vi "PAM v1.3.vi"() -> ()   [LabVIEW 2011]
uses:
  PAM_Control.ctl
  <vilib>/Utility/error.llb/DialogType.ctl
  <vilib>/Analysis/Matrix/Datatypes/RealMatrix.ctl
  <vilib>/DAQmx/read.llb/DAQmx Read (Analog 1D Wfm NChan NSamp).vi
  <vilib>/DAQmx/write.llb/DAQmx Write (Analog 1D DBL NChan 1Samp).vi
  PAM SubVIs/RH Probe Global Var.vi
  <vilib>/DAQmx/configure/timing.llb/DAQmx Timing (Sample Clock).vi
  <vilib>/Utility/file.llb/Write To Spreadsheet File (string).vi
  <vilib>/Analysis/Matrix/Numeric/Conversions/Matrix To Array - RM.vi
  <vilib>/DAQmx/miscellaneous.llb/DAQmx Fill In Error Info.vi
  Program Files (x86)/National Instruments/LabVIEW 2011/resource/objmgr/daqmx.rc
  <vilib>/Analysis/Matrix/NI_Matrix.lvlib
panel:
  out "O3 Data":sgl[](graph)
  out "SO2 Data":sgl[](graph)
  out "NO, NO2, NOx Data":dbl[][](graph)
  out "Bad Advantech Data Points":dbl
  out "Run In Progress?":bool
  out "Manual":bool
  in  "MFC Sequence File":path=path "C:/Users/PAM/Dropbox/Research - Dr. Williams/PAM/LabVIEW PAM/PAM Edited/defaultMFCSequence.txt"
  out "Auto":bool
  out "P Unit":string
  out "Pressure Transducer":dbl(knob) scale=1.0004682058141296e-16..9998.829827870512
  out "Error Out":errorcluster
  out "Elapsed Time (min)":dbl format="%#_2g"
  in  "Run Start Time":timestamp format="%<%X\n%x>T"
  out "NOx Units":string="LPM"
  in  "NOx Control (LPM)":dbl(slide) scale=0.0..0.5
  out "NOx Reading (LPM) 3":dbl(slide) scale=0.0..0.5
  out "VOC Units":string="LPM"
  in  "VOC Control (LPM)":dbl(slide) scale=0.0..0.04
  out "VOC Reading (LPM)":dbl(slide) scale=0.0..0.04
  out "O2 Units":string="LPM"
  in  "O2 Control (LPM)":dbl(slide) scale=0.0..1.0
  out "O2 Reading (LPM)":dbl(slide) scale=0.0..1.0 scale format="%#.2f"
  out "N2 Units":string="LPM"
  in  "N2 Control (LPM)":dbl(slide) scale=0.0..20.0
  out "N2 Reading (LPM)":dbl(slide) scale=0.0..20.0 scale format="%#.2f"
  out "AI (non TC) Units":string[](array[string])
  out "AI (non TC) Names":string[](array[string])
  out "RH Values":dbl[](array[numeric]) format="%#.2f"
  out "All Temp Units":i32[](array[ring]) items=["Deg C"=10143, "Deg F"=10144, "Kelvins"=10325, "Deg R"=10145, "From Custom Scale"=10065]
  out "All TC Labels":string[](array[string])
  out "TC Values Readings":dbl[](array[numeric]) format="%#_3g"
  out "Relative Humidity Data":waveform(dbl)[](graph) caption="Waveform Chart"
  in  "Stop Button":bool
  out "Temperature Data":dynamicdata(graph) caption="Waveform Chart"
  in  "Sampling Frequency (Hz)":dbl=5.0 caption="Delay Time (s)"
  in  "Trigger Type":T1(tab)
  in  "In Use? 11":bool=TRUE
  in  "In Use? 10":bool=TRUE
  in  "In Use? 9":bool=TRUE
  in  "In Use? 8":bool=TRUE
  in  "In Use? 7":bool=TRUE
  in  "In Use? 6":bool=TRUE
  in  "In Use? 5":bool=TRUE
  in  "Adv. TC 7":string="TC 7"
  in  "Adv. TC 6":string="TC 6"
  in  "Adv. TC 5":string="TC 5"
  in  "Adv. TC 4":string="TC 4"
  in  "Adv. TC 3":string="TC 3"
  in  "Adv. TC 2":string="TC 2"
  in  "Adv. TC 1":string="TC 1"
  in  "units":i32(ring)=10143 items=["Deg C"=10143, "Deg F"=10144, "Kelvins"=10325, "Deg R"=10145, "From Custom Scale"=10065]
  in  "In Use? 14":bool=TRUE
  in  "Physical Channel 14":tag="Dev1/ai7"
  in  "TC 14":string="PAM Downstream T"
  in  "In Use? 13":bool=TRUE
  in  "Physical Channel 13":tag="Dev1/ai3"
  in  "TC 13":string="Humidifier T"
  in  "In Use? 12":bool
  in  "Physical Channel 12":tag="Dev1/ai23"
  in  "TC 12":string="TC 12"
  in  "In Use? 15":bool
  in  "In Use? 14":bool
  in  "In Use? 13":bool
  in  "In Use? 12":bool
  in  "Physical Channel 4":tag="Dev1/ai21"
  in  "TC 4":string="TC 11"
  in  "Physical Channel 3":tag="Dev1/ai17"
  in  "TC 3":string="TC 10"
  in  "Physical Channel 2":tag="Dev1/ai20"
  in  "TC 2":string="TC 9"
  in  "Physical Channel":tag="Dev1/ai16"
  in  "TC 1":string="TC 8"
  in  "Thermocouple Type 1":T2=10073 items=["J"=10072, "K"=10073, "N"=10077, "R"=10082, "S"=10085, "T"=10086, "B"=10047, "E"=10055]
  in  "Min Value (deg C)":dbl
  in  "Max Value (deg C)":dbl=100.0
  in  "CJC Source":i32(ring)=10116 items=["Built-In"=10200, "Constant Value"=10116, "Channel"=10113]
  in  "CJC Value":dbl=25.0 format="%0.2f"
  in  "CJC Channel":refnum<k21>
  in  "In Use? 3":bool=TRUE
  in  "In Use? 4":bool=TRUE
  in  "RHT  2":tag="Dev1/ai5"
  in  "RHT Probe 2":string="RH 2"
  in  "RHT  1":tag="Dev1/ai4"
  in  "RHT Probe 1":string="RH 1"
  in  "In Use? 1":bool=TRUE
  in  "RHT  4":tag="Dev1/ai1"
  in  "RHT Probe 4":string="RHT T2"
  in  "RHT  3":tag="Dev1/ai0"
  in  "RHT Probe 3":string="RHT T1"
  in  "In Use? 2":bool=TRUE
  in  "Vaisala RH Scale":tag="RH Vaisala"
  in  "Vaisala T Scale":tag="RHT - Temp"
  in  "physical channels 4":tag="Dev1/ao3"
  out "Scale for VOC MFC 2":tag="NOx uMFC B"
  out "VOC MFC 2":string="VOC"
  in  "physical channels 3":tag="Dev1/ao2"
  out "Scale for NOx MFC 2":tag="NOx uMFC A"
  out "NOx MFC 2":string="NOx"
  in  "physical channels 2":tag="Dev1/ao1"
  out "Scale for O2 MFC 2":tag="O2 MFC B"
  out "O2 MFC 2":string="O2"
  in  "Scale for VOC MFC":tag="NOx uMFC B"
  in  "VOC MFC Channel":tag="Dev1/ai22"
  in  "VOC MFC":string="VOC"
  in  "Scale for NOx MFC":tag="NOx uMFC A"
  in  "NOx MFC Channel":tag="Dev1/ai18"
  in  "NOx MFC":string="NOx"
  in  "Scale for O2 MFC":tag="O2 MFC B"
  in  "O2 MFC Channel":tag="Dev1/ai6"
  in  "O2 MFC":string="O2"
  in  "Scale for N2 MFC":tag="N2 MFC A"
  in  "N2 MFC Channel":tag="Dev1/ai2"
  in  "N2 MFC":string="N2"
  out "Scale for N2 MFC 2":tag="N2 MFC A"
  out "N2 MFC 2":string="N2"
  in  "physical channels":tag="Dev1/ao0"
  in  "Units":enum16{"Torr", "Psia", "Bar", "kPa"}(ring)
  in  "In Use? 16":bool=TRUE
  in  "Pressure Transducer Channel":tag="Dev1/ai19"
  in  "Pressure Transducer Label":string="Pressure"
  in  "In Use? 18":bool=TRUE
  in  "Instrument 3":T3(ring)=enum."O3 (49i)"
  in  "In Use? 17":bool=TRUE
  in  "Instrument 2":T3(ring)=enum."SO2 (43i-TLE)"
  in  "In Use? 17":bool=TRUE
  in  "Instrument":T3(ring)
  in  "Frequency (Hz)":dbl=0.1
  in  "Log Thermo Data?":bool
  out "File Path for Gas Analyzer Data":string
  out "File Path for PAM Data":string
  in  "Header Information":string[][](array[string])
  in  "Delimeter":string="\t"
  in  "Log PAM Data?":bool
  in  "folder path for Data (dialog if empty) 2":path=path "C:/Users/PAM/Documents/PAM DATA/Data Auto"
  in  "Data Logging Interval (s)":dbl=2.0 caption="Delay Time (s)"
  # "Timing Settings"
  # "DAQ Setup & More"
  # "NOx MFC controls and indicators"
  # "VOC MFC controls and indicators"
  # "O2 MFC controls and indicators"
  # "N2 MFC controls and indicators"
  # "Analog Input (non TC) Readings"
  # "Thermocouple Readings"
  # "Currently Out Of Order :/"
  # "TC 1"
  # "Advantech ai0"
  # "TC 2"
  # "Advantech ai1"
  # "TC 3"
  # "Advantech ai2"
  # "TC 4"
  # "Advantech ai3"
  # "TC 5"
  # "Advantech ai4"
  # "TC 6"
  # "Advantech ai5"
  # "TC 7"
  # "Advantech ai6"
  # "TC 8"
  # "TC 9"
  # "TC 10"
  # "TC 11"
  # "TC 12"
  # "TC 13"
  # "TC 14"
  # "Vaisala RHT Probe (RH Settings)"
  # "Vaisala RHT Probe (Temp. Settings)"
  # "MFC Analog Input Setup"
  # "MFC Analog Ouput Setup"
  # "VOC MFC"
  # "NOx MFC"
  # "O2 MFC"
  # "VOC MFC"
  # "NOx MFC"
  # "O2 MFC"
  # "N2 MFC"
  # "N2 MFC"
  # "O3 [Model 49i]"
  # "SO2 [Model 43i-TLE]"
  # "NO, NO2, NOx [Model 42i-TL]"
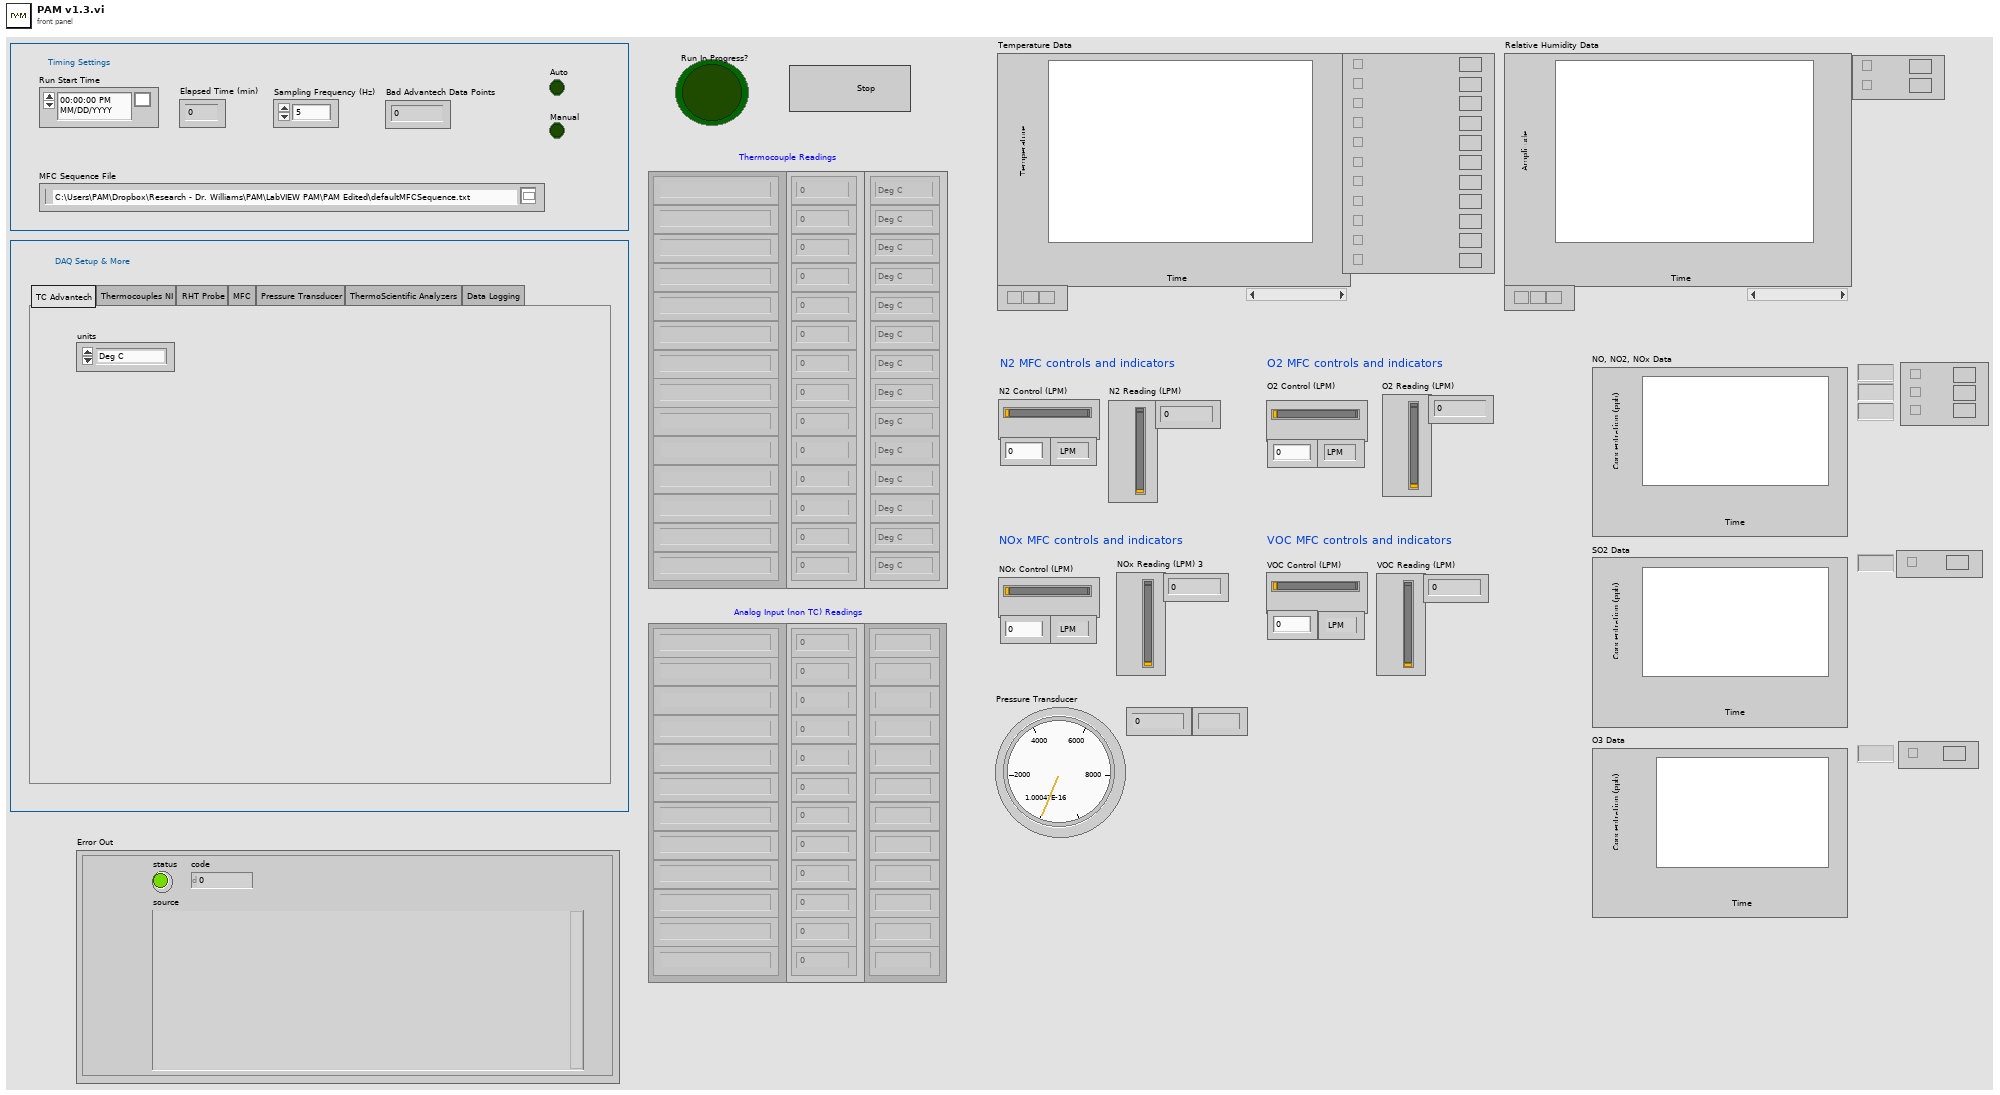
[diagram p1: front panel]
types:
  T1 = enum32{"TC Advantech", "Thermocouples NI", "RHT Probe", "MFC", "Pressure Transducer", "ThermoScientific Analyzers", "Data Logging"}
  T2 = typedef "PAM_Control.ctl" = i32
  T3 = enum16{"NOx (42i-TL)", "SO2 (43i-TLE)", "O3 (49i)"}
  T4 = cluster{"Label":string, "Boolean":bool, "Channel":tag, "Units":string, "Units Num":i32}[]
  T5 = cluster{"Label":string, "Channel":tag, "Scale":tag}[]
  T6 = cluster{"Label":string, "SP N2":dbl, "Time":dbl, "SP O2":dbl, "SP NOx":dbl, "SP VOC":dbl}[]
  T7 = typedef "NI_Matrix.lvlib/RealMatrix.ctl" = dbl[][]
  T8 = typedef "DialogType.ctl" = u16
  T9 = cluster{"Label":string, "Concentration":sgl, "Units":string}[]
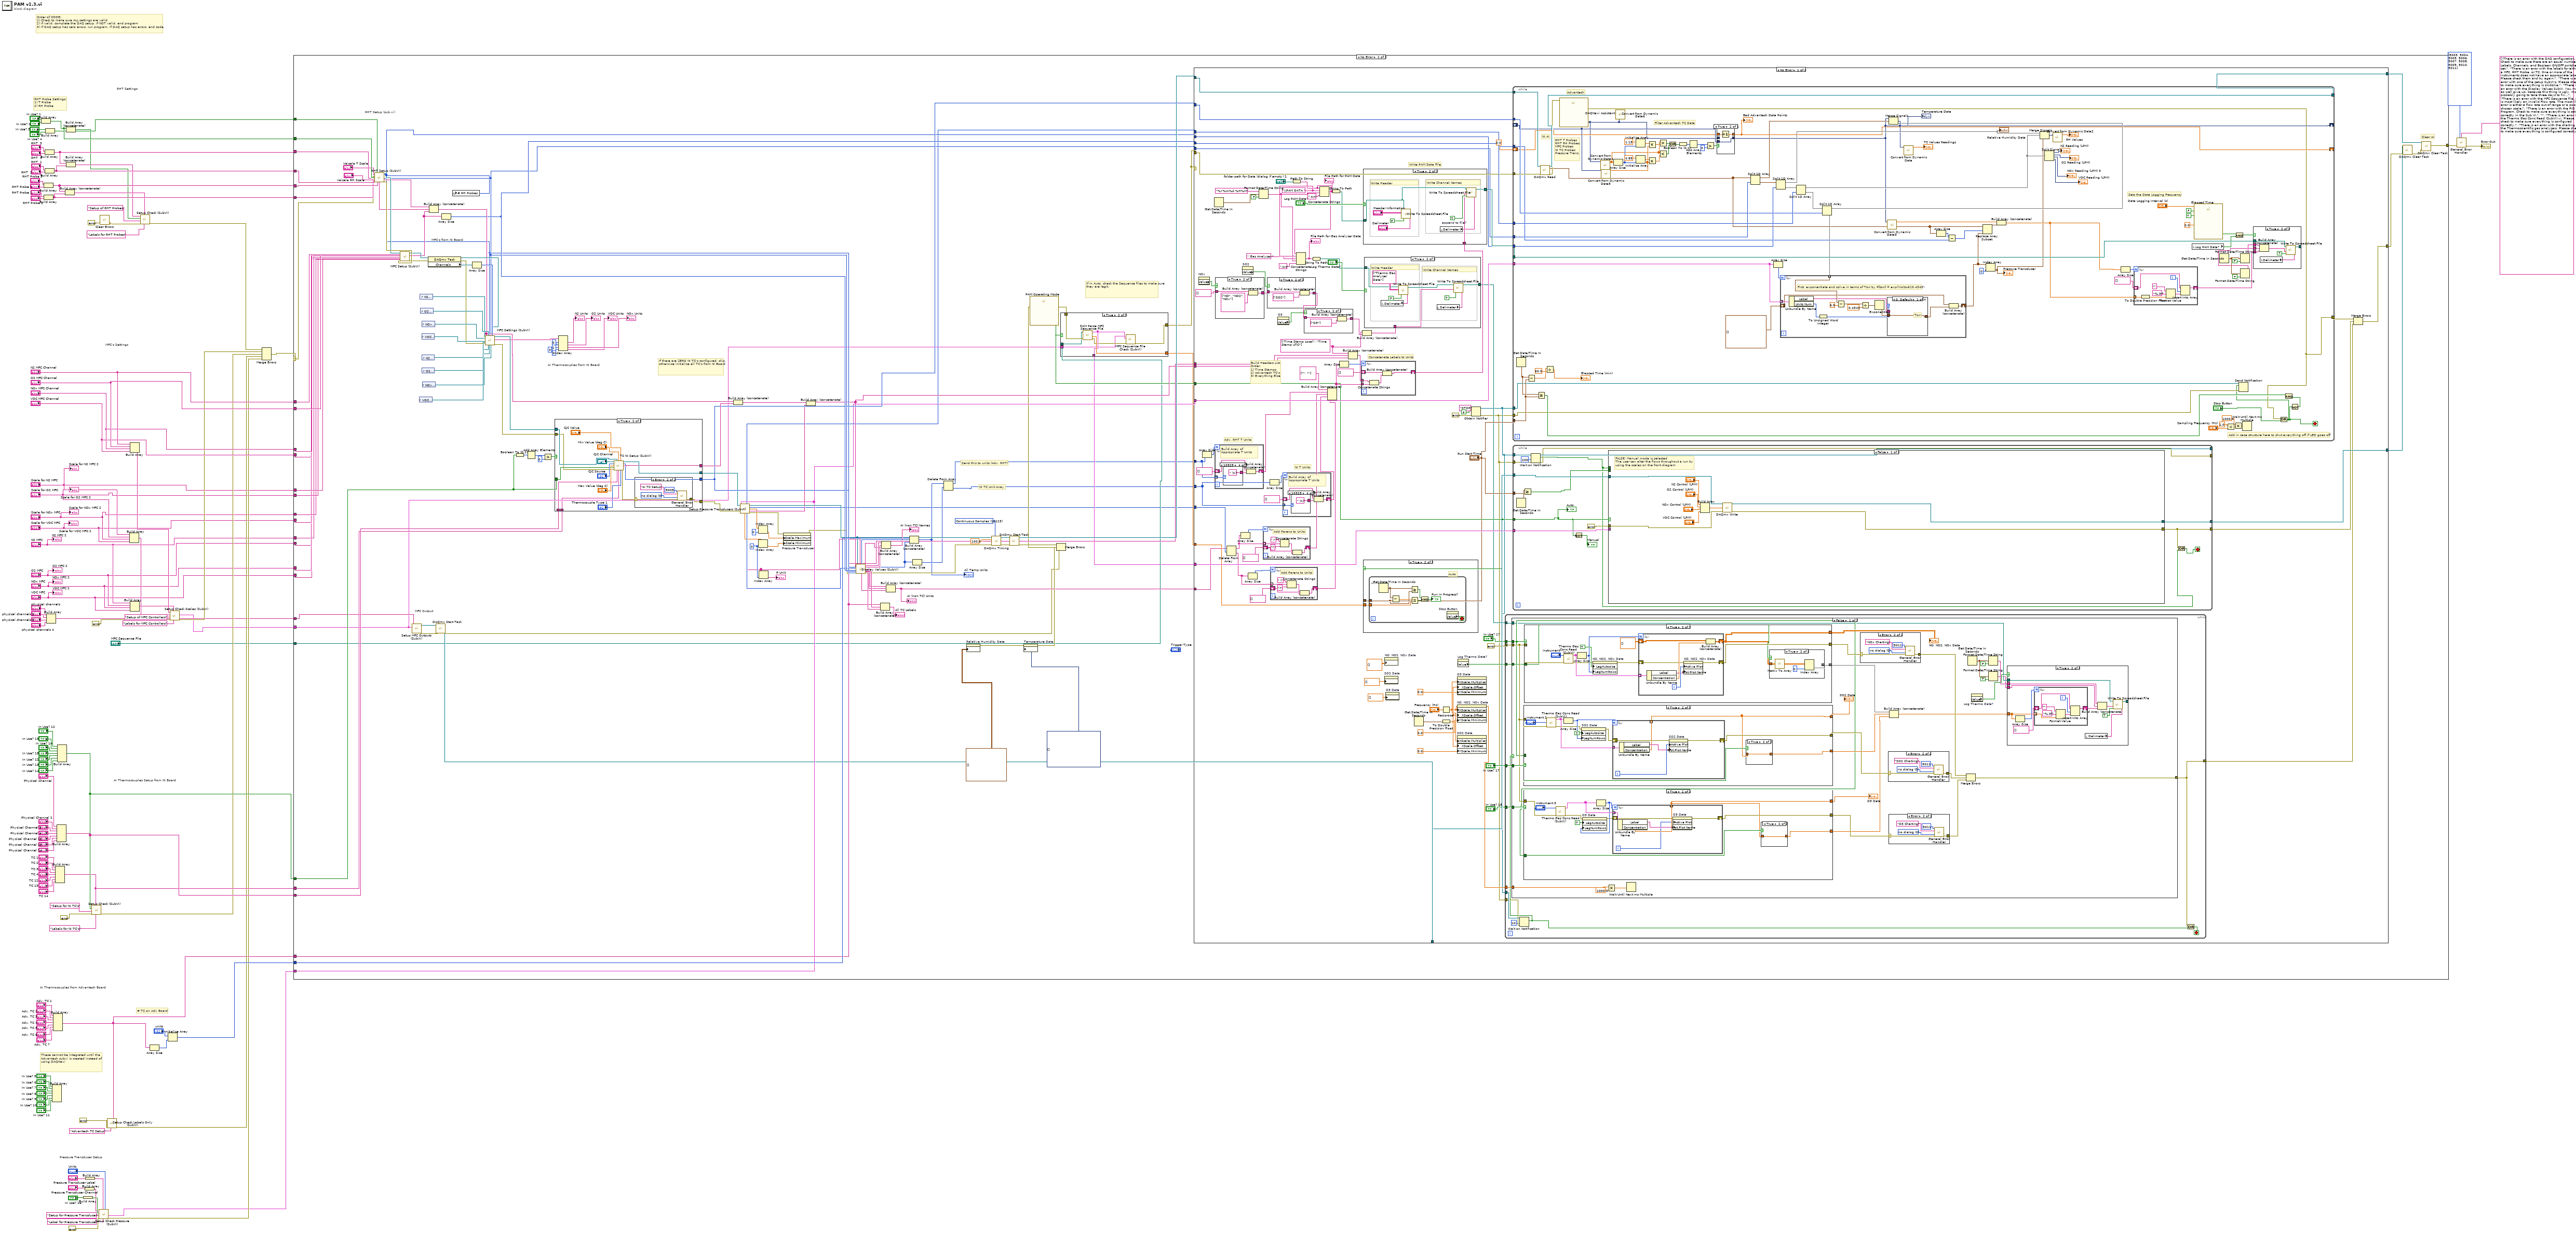
[diagram p0: block diagram]
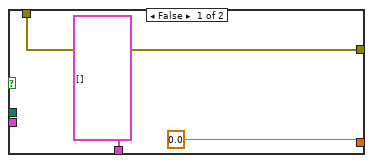
[diagram p2: hidden frame]
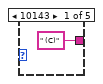
[diagram p3: hidden frame]
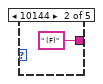
[diagram p4: hidden frame]
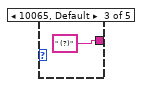
[diagram p5: hidden frame]
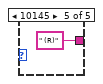
[diagram p6: hidden frame]
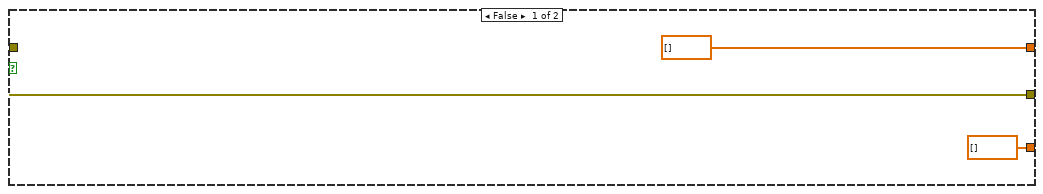
[diagram p15: hidden frame]
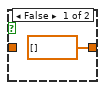
[diagram p16: hidden frame]
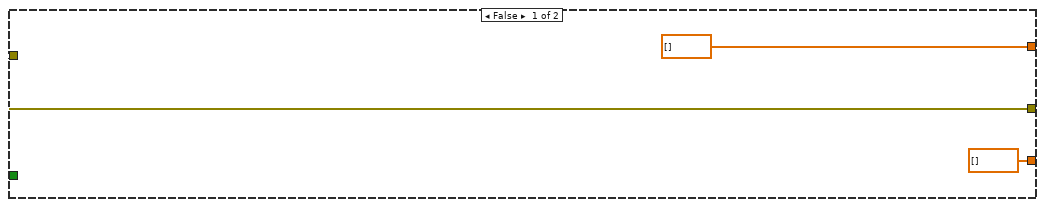
[diagram p17: hidden frame]
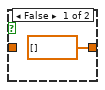
[diagram p18: hidden frame]
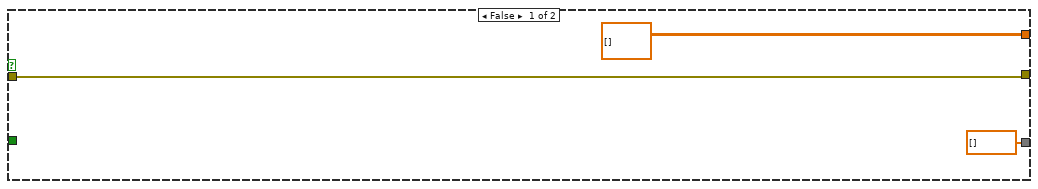
[diagram p19: hidden frame]
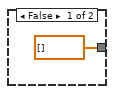
[diagram p20: hidden frame]
diagram:
  # "Pressure Transducer Setup"
  # "AI Thermocouples Setup from NI Board"
  # "MFC's Settings"
  # "Order of CODE:\n1) Check to make sure ALL settings are valid\n2) If valid, complete the DAQ setup. If NOT valid, end program\n3) If DAQ setup has zero errors, run program. If DAQ setup has errors, end code."
  # "RHT Probe Settings:\n1) T Probe\n2) RH Probe"
  # "These cannot be integrated until the Advantech subvi is created instead of using DAQNavi"
  # "RHT Settings"
  # "# TC on Adv Board"
  # "AI Thermocouples from Advantech Board"
  n1 = Build Array("In Use? 1", "In Use? 2") -> (w71:bool[])
  n2 = Build Array("RHT Probe 3", "RHT Probe 4") -> (w67:string[])
  n3 = Build Array("RHT Probe 1", "RHT Probe 2") -> (w66:string[])
  n4 = Build Array("RHT  3", "RHT  4") -> (w69:tag[])
  n5 = Build Array("RHT  1", "RHT  2") -> (w68:tag[])
  n6 = Build Array("In Use? 3", "In Use? 4") -> (w70:bool[])
  n7 = Build Array("physical channels", "physical channels 2", "physical channels 3", "physical channels 4") -> (w3:tag[])
  n8 = Build Array("In Use? 5", "In Use? 6", "In Use? 7", "In Use? 8", "In Use? 9", "In Use? 10", "In Use? 11") -> ()  [unwired: 1 out]
  n9 = Build Array("Adv. TC 1", "Adv. TC 2", "Adv. TC 3", "Adv. TC 4", "Adv. TC 5", "Adv. TC 6", "Adv. TC 7") -> (w38:string[])
  n10 = Build Array("TC 1", "TC 2", "TC 3", "TC 4", "TC 12", "TC 13", "TC 14") -> (w50:string[])
  n11 = Build Array("Physical Channel", "Physical Channel 2", "Physical Channel 3", "Physical Channel 4", "Physical Channel 12", "Physical Channel 13", "Physical Channel 14") -> (w51:tag[])
  n12 = Build Array("In Use? 12", "In Use? 13", "In Use? 14", "In Use? 15", "In Use? 12", "In Use? 13", "In Use? 14") -> (w52:bool[])
  n13 = Build Array (concatenate)(w67, w66) -> (w65:string[])
  n14 = Build Array (concatenate)(w69, w68) -> (w42:tag[])
  n15 = Build Array (concatenate)(w71, w70) -> (w41:bool[])
  n16 = Build Array("In Use? 16") -> (w32:bool[])
  n17 = Build Array("Pressure Transducer Channel") -> (w31:tag[])
  n18 = Build Array("Pressure Transducer Label") -> (w33:string[])
  n19 = call "Setup Check (SubVI).vi"("[error source] (\" \")"="Labels for NI TC's" ("[error source] (\" \")"), "Labels Array"=w50, "error in (no error)"=errorcluster {"status"=FALSE, "code"=0, "source"=""} ("error constant"), "[error source] (\" \") 2"="Setup for NI TC's" ("[error source] (\" \") 2"), "Boolean Array"=w52, "Channel Array"=w51) -> ("error out"=w46:errorcluster)  [unwired: 4 in, 1 out]
  n20 = call "Setup Check Pressure (SubVI).vi"("Units"="Units", "[error source] (\" \")"="Label for Pressure Transducer" ("[error source] (\" \")"), "Labels Array"=w33, "error in (no error)"=errorcluster {"status"=FALSE, "code"=0, "source"=""} ("error constant"), "[error source] (\" \") 2"="Setup for Pressure Transducer" ("[error source] (\" \") 2"), "Boolean Array"=w32, "Channel Array"=w31) -> ("error out"=w27:errorcluster, "Cluster Out"=w25:T4)  [unwired: 3 in]
  n21 = call <vilib>:"Clear Errors.vi"("error in (no error)"=errorcluster {"status"=FALSE, "code"=0, "source"=""} ("error constant")) -> ("error out"=w73:errorcluster)  [unwired: 6 in]
  n22 = call "Setup Check Labels Only (SubVI).vi"("error in (no error)"=errorcluster {"status"=FALSE, "code"=0, "source"=""} ("error constant"), "[error source] (\" \")"="Advantech TC Setup" ("[error source] (\" \")"), "Labels Array"=w38) -> ("error out"=w44:errorcluster)  [unwired: 6 in, 1 out]
  n23 = Build Array("Scale for N2 MFC", "Scale for O2 MFC", "Scale for NOx MFC", "Scale for VOC MFC") -> (w56:tag[])
  n24 = Build Array("N2 MFC Channel", "O2 MFC Channel", "NOx MFC Channel", "VOC MFC Channel") -> (w59:tag[])
  n25 = Build Array("N2 MFC", "O2 MFC", "NOx MFC", "VOC MFC") -> (w57:string[])
  n26 = call "Setup Check (SubVI).vi"("[error source] (\" \")"="Labels for RHT Probes" ("[error source] (\" \")"), "Labels Array"=w65, "error in (no error)"=w73, "[error source] (\" \") 2"="Setup of RHT Probes" ("[error source] (\" \")"), "Boolean Array"=w41, "Channel Array"=w42) -> ("error out"=w64:errorcluster)  [unwired: 4 in, 1 out]
  n27 = Array Size(array=w38) -> (size(s)=w102:i32)
  n28 = Initialize Array("units", w102) -> (w101:i32[])
  n29 = call "Setup Check Scales (SubVI).vi"("[error source] (\" \")"="Labels for MFC Controllers" ("[error source] (\" \")"), "Labels Array"=w57, "error in (no error)"=errorcluster {"status"=FALSE, "code"=0, "source"=""} ("error constant"), "[error source] (\" \") 2"="Setup of MFC Controllers" ("[error source] (\" \") 2"), "Scale Array"=w56, "Channel Array"=w59) -> ("error out"=w53:errorcluster, "Array of Clusters Out"=w2:T5)  [unwired: 4 in]
  n30 = Merge Errors(w64, w53, w46, w44, w27) -> (w39:errorcluster)
  n31 = case shown="No Error" w39 {
    selector: w39 -> [w152 w901]
    tunnel: w101 -> [w220 _]
    tunnel: [w203 w901] -> w89
    tunnel: w71 -> [w202 _]
    tunnel: w70 -> [w201 _]
    tunnel: w69 -> [w200 _]
    tunnel: w68 -> [w199 _]
    tunnel: w67 -> [w198 _]
    tunnel: w66 -> [w197 _]
    tunnel: "N2 MFC Channel" -> [w194 _]
    tunnel: "O2 MFC Channel" -> [w193 _]
    tunnel: "NOx MFC Channel" -> [w192 _]
    tunnel: "VOC MFC Channel" -> [w191 _]
    tunnel: "Scale for N2 MFC" -> [w190 _]
    tunnel: "Scale for O2 MFC" -> [w189 _]
    tunnel: "Scale for NOx MFC" -> [w188 _]
    tunnel: "Scale for VOC MFC" -> [w187 _]
    tunnel: "N2 MFC" -> [w186 _]
    tunnel: "O2 MFC" -> [w185 _]
    tunnel: "NOx MFC" -> [w184 _]
    tunnel: "VOC MFC" -> [w183 _]
    tunnel: w52 -> [w181 _]
    tunnel: w51 -> [w180 _]
    tunnel: w50 -> [w179 _]
    tunnel: w38 -> [w178 _]
    tunnel: w25 -> [w164 _]
    tunnel: w3 -> [w151 _]
    tunnel: w2 -> [w128 _]
    tunnel: "MFC Sequence File" -> [w131 _]
    frame No Error {
      w156 = 0 ("index")
      w209 = 10123 items=["Finite Samples"=10178, "Continuous Samples"=10123, "Hardware Timed Single Point"=12522] ("sample mode")
      # "NI TC Unit Array"
      # "Send this to units (Adv, RHT)"
      # "If in Auto, check the Sequence files to make sure they are legit."
      # "MFC Output"
      # "RHT Setup (sub.vi)"
      # "If there are ZERO NI TC's configured, skip, otherwise initialize all TC's from NI Board"
      # "Clear AI"
      # "MFC's from NI Board"
      # "AI Thermocouples from NI Board"
      n32 = call "RHT Setup (SubVI).vi"("RH Used?"=w201, "Vaisala T Scale"="Vaisala T Scale", "Error In"=w152, "TC Used?"=w202, "RHT (T) Channels"=w200, "Vaisala RH Scale"="Vaisala RH Scale", "RH Names"=w197, "RH Channels"=w199, "RHT (T) Names"=w198) -> ("RH Labels"=w234:string[], "Refnum out"=w244:refnum<k21>, "# RH Probes"=w204:i32, "# RH (T) Probes"=w205:i32, "RH (T) Labels"=w237:string[], "error out"=w245:errorcluster)  [unwired: 13 in]
      n33 = call "MFC Setup (SubVI).vi"("Refnum in"=w244, "O2 MFC"=w185, "VOC MFC Channel"=w191, "Scale for VOC MFC"=w187, "NOx MFC"=w184, "error in (no error)"=w245, "NOx MFC Channel"=w192, "VOC MFC"=w183, "N2 MFC"=w186, "Scale for N2 MFC"=w190, "O2 MFC Channel"=w193, "Scale for O2 MFC"=w189, "N2 MFC Channel"=w194, "Scale for NOx MFC"=w188) -> ("Refnum out"=w242:refnum<k21>, "Array"=w218:string[], "error out"=w241:errorcluster)  [unwired: 3 in]
      n34 = call "Setup MFC Outputs (SubVI).vi"("Array of Clusters In"=w128, "Array"=w151) -> ("error out"=w147:errorcluster, "Refnum out"=w144:refnum<k21>)  [unwired: 8 in]
      n35 = control-ref of="VOC Control (LPM)"() -> (w222:refnum<vi>)
      n36 = control-ref of="N2 Reading (LPM)"() -> (w119:refnum<vi>)
      n37 = control-ref of="O2 Reading (LPM)"() -> (w226:refnum<vi>)
      n38 = control-ref of="VOC Reading (LPM)"() -> (w182:refnum<vi>)
      n39 = control-ref of="N2 Control (LPM)"() -> (w224:refnum<vi>)
      n40 = control-ref of="O2 Control (LPM)"() -> (w223:refnum<vi>)
      n41 = control-ref of="NOx Reading (LPM) 3"() -> (w225:refnum<vi>)
      n42 = control-ref of="NOx Control (LPM)"() -> (w221:refnum<vi>)
      n43 = property class="DAQmx Task"(reference=w242, error in=w241) -> (reference out=w239:refnum<k21>, error out=w146:errorcluster, "Channels"=w238:refnum<k21>[])
      n44 = Build Array (concatenate)(w237, w234, w218) -> (w219:string[])
      n45 = call <vilib>:"DAQmx Start Task.vi"("task/channels in"=w144, "error in"=w147) -> ("task out"=w150:refnum<k21>, "error out"=w149:errorcluster)  [unwired: 12 in]
      n46 = Array Size(array=w218) -> (size(s)=w217:i32)
      n47 = global write "RH Probe Global Var.vi" "# RH Probes"(w204) -> ()
      n48 = Array Size(array=w238) -> (size(s)=w243:i32)
      n49 = call "MFC Settings (SubVI).vi"("N2 Control"=w119, "NOx Control"=w225, "Channel Names"=w219, "VOC Control"=w182, "N2 Display"=w224, "error in (no error)"=w146, "O2 Control"=w226, "O2 Display"=w223, "# RH Probes"=w204, "VOC Display"=w222, "# RH (T) Probes"=w205, "NOx Display"=w221, "# Channels"=w243, "task in"=w239) -> ("Refnum out"=w240:refnum<k21>, "MFC Units"=w143:string[], "error out"=w213:errorcluster)  [unwired: 3 in]
      n50 = Boolean To (0,1)(Boolean=w181) -> (0, 1=w214:i16[])
      n51 = Add Array Elements(numeric array=w214) -> (sum=w212:i16)
      n52 = Greater?(x=w212, y=i16 0) -> (0:w210:bool)
      n53 = case shown="True" w210 {
        tunnel: [w877 w879] -> w165
        tunnel: w240 -> [w878 w888]
        tunnel: [w878 w887] -> w173
        tunnel: w180 -> [_ w886]
        tunnel: w179 -> [_ w885]
        tunnel: [string[] [] ("Labels") w884] -> w216
        tunnel: [0 ("# TC (NI)") w883] -> w215
        tunnel: w181 -> [_ w882]
        tunnel: w213 -> [w877 w881]
        frame False {
        }
        frame True {
          n54 = call "TC NI Setup (SubVI).vi"("Refnum in"="CJC Channel", "Refnum out"=w888, "Min Value (deg C)"="Min Value (deg C)", "CJC Value"="CJC Value", "CJC Source"="CJC Source", "Max Value (deg C)"="Max Value (deg C)", "Boolean Array In"=w882, "error in (no error)"=w881, "Physical Channels"=w886, "Labels In"=w885, "Thermocouple Type 1"="Thermocouple Type 1") -> ("Refnum out"=w887:refnum<k21>, "# TC (NI)"=w883:i32, "Labels"=w884:string[], "error out"=w880:errorcluster)  [unwired: 1 in]
          n55 = case shown="Error" w880 {
            selector: w880 -> [w895 w899]
            tunnel: [w895 w900] -> w879
            frame No Error {
            }
            frame Error {
              w897 = T8 0 items=["no dialog", "OK message", "continue or stop message", "OK message + warnings", "continue/stop + warnings"] ("type of dialog (OK msg:1)")
              n56 = call <vilib>:"General Error Handler.vi"("[error code] (0)"=5005, "[error source] (\" \")"="AI TC Setup" ("[error source] (\" \")"), "type of dialog (OK msg:1)"=w897, "error in (no error)"=w899) -> ("error out"=w900:errorcluster)  [unwired: 7 in, 4 out]
            }
          }
        }
      }
      n57 = Index Array(array=w143, index #1=0 ("index"), index #2=1 ("index"), index #3=2 ("index"), index #4=3 ("index")) -> (element #1=→"N2 Units":string, element #2=→"O2 Units":string, element #3=→"NOx Units":string, element #4=→"VOC Units":string)
      n58 = Build Array (concatenate)(w219, w216) -> (w168:string[])
      n59 = call "Setup Pressure Transducers (SubVI).vi"("Refnum in"=w173, "Cluster Out"=w164, "Error In"=w165) -> ("Units"=w155:string[], "Refnum out"=w172:refnum<k21>, "# PT"=w120:i32, "Max Out"=w161:dbl[], "Array"=w169:string[], "Min Out"=w163:dbl[], "# Pressure Transducers"=w166:i32, "Error Out"=w159:errorcluster)  [unwired: 4 in, 1 out]
      n60 = Index Array(array=w161, index=0) -> (element=w158:dbl)
      n61 = Index Array(array=w163, index=w156) -> (element=w157:dbl)
      n62 = Index Array(array=w155, index=w156) -> (element=→"P Unit":string)
      n63 = property on="Pressure Transducer" class="Knob (strict)"(error in=w159, "Scale.Maximum"=w158, "Scale.Minimum"=w157) -> (error out=w160:errorcluster)  [unwired: 1 in, 1 out]
      n64 = Build Array (concatenate)(w168, w169) -> (w167:string[])
      n65 = call "Display Values (SubVI).vi"("Channels List"=w172, "All Names"=w167, "# PT"=w166, "# MFC"=w217, "# RH (T) Probes"=w205, "error In"=w160, "# TC (NI)"=w215, "# RH Probes"=w204, "PT Units In"=w155) -> ("NI TC Names"=w233:string[], "RH (T) Units"=w232:i32[], "PT Units Out"=w170:string[], "NI TC Units"=w125:i32[], "RH (T) Names"=w236:string[], "RH Names"=w230:string[], "MFC Names"=w228:string[], "PT Names"=w171:string[], "RH Units"=w229:string[], "MFC Units"=w227:string[], "error out"=w177:errorcluster)
      n66 = Build Array (concatenate)(w178, w236, w233) -> (→"All TC Labels":string[])
      n67 = Build Array (concatenate)(w230, w228, w171) -> (→"AI (non TC) Names":string[])
      n68 = Build Array (concatenate)(w229, w227, w170) -> (w153:string[])
      "AI (non TC) Units" <- w153
      n69 = Build Array (concatenate)(w220, w232, w125) -> (w122:i32[])
      "All Temp Units" <- w122
      n70 = Array Size(array=w125) -> (size(s)=w124:i32)
      n71 = Delete From Array(array=w122, length=w124) -> (deleted portion=w121:i32[], array with subset deleted=w123:i32[])  [unwired: 1 in]
      n72 = property on="Relative Humidity Data" class="WFChart (strict)"("History Data"=waveform(dbl)[][] []) -> (error out=w247:errorcluster)  [unwired: 2 in, 1 out]
      n73 = call-poly <vilib>:"DAQmx Timing.vi"("task/channels in"=w172, "sample mode"=w209, "rate"=100.0, "error in"=w177) -> ("task out"=w207:refnum<k21>, "error out"=w176:errorcluster)  [unwired: 10 in]
      n74 = call <vilib>:"DAQmx Start Task.vi"("task/channels in"=w207, "error in"=w176) -> ("task out"=w206:refnum<k21>, "error out"=w175:errorcluster)  [unwired: 12 in]
      n75 = property on="Temperature Data" class="WFChart (strict)"(error in=w247, "History Data"=dynamicdata[] []) -> (error out=w246:errorcluster)  [unwired: 1 in, 1 out]
      n76 = Merge Errors(w175, w246, w149) -> (w145:errorcluster)
      n77 = call "PAM Operating Mode"("error in (no error)"=w145) -> ("Auto"=w134:bool, "error out"=w133:errorcluster)  [unwired: 17 in]
      n78 = case shown="True" w134 {
        tunnel: w133 -> [w252 w259]
        tunnel: [w252 w253] -> w132
        tunnel: w131 -> [_ w258]
        tunnel: [T6 [] ("Cluster Out") w256] -> w130
        tunnel: [0.0 ("Time (Last)") w257] -> w129
        tunnel: w128 -> [_ w254]
        frame False {
        }
        frame True {
          n79 = call "PAM Parse MFC Sequence File.vi"("error in"=w259, "Sequence File"=w258) -> ("error out"=w255:errorcluster, "Time (Last)"=w257:dbl, "Cluster Out"=w256:T6)  [unwired: 7 in]
          n80 = call "MFC Sequence File Check (SubVI).vi"("error in (no error)"=w255, "Sequence Cluster"=w256, "Cluster of MFCs"=w254) -> ("error in (no error) 2"=w253:errorcluster)  [unwired: 8 in]
        }
      }
      n81 = case shown="No Error" w132 {
        tunnel: w217 -> [w344 _]
        tunnel: w215 -> [w343 _]
        tunnel: w167 -> [w342 _]
        tunnel: w132 -> [w341 w874]
        tunnel: w206 -> [w340 w873]
        tunnel: w205 -> [w339 _]
        tunnel: w204 -> [w338 _]
        tunnel: w178 -> [w337 _]
        tunnel: [w336 w873] -> w174
        tunnel: [w317 w874] -> w127
        tunnel: w166 -> [w335 _]
        tunnel: w164 -> [w334 _]
        tunnel: w123 -> [w332 _]
        tunnel: w153 -> [w265 _]
        tunnel: w150 -> [w320 w872]
        tunnel: [w319 w872] -> w126
        tunnel: w134 -> [w314 _]
        tunnel: w130 -> [w315 _]
        tunnel: w129 -> [w312 _]
        tunnel: w121 -> [w268 _]
        tunnel: w120 -> [w266 _]
        frame No Error {
          w295 = "\\PAM DATA " ("string")
          w276 = string[] ["Time Stamp Local", "Time Stamp UTC"] ("array")
          # "NI T Units"
          # "Adv, RHT T Units"
          # "Write PAM Data File"
          # "Concatenate Labels to Units"
          # "Build Headers List \nOrder:\n1) Time Stamps\n2) Advantech TC's\n3) Everything Else"
          n82 = property on="NOx" class="Bool (strict)"() -> ("Value"=w287:bool)  [unwired: 2 in, 2 out]
          n83 = Array Size(array=w332) -> (size(s)=w333:i32)
          n84 = Get Date/Time In Seconds() -> (seconds since 1Jan1904=w350:timestamp)
          n85 = for {
            N: w333 -> [_]
            tunnel: w332 -> [w721] mode=indexing
            shift-right: [w720] -> w329
            shift-left: string[] [] -> [w718]
            # "Build Array of Appropriate T Units"
            n86 = case shown="10325" w721 {
              tunnel: [" (C)" " (F)" " (?)" " (K)" " (R)"] -> w719
              frame 10143 {
              }
              frame 10144 {
              }
              frame 10065, Default {
              }
              frame 10325 {
              }
              frame 10145 {
              }
            }
            n87 = Build Array (concatenate)(w718, w719) -> (w720:string[])
          }
          n88 = case shown="True" w287 {
            tunnel: [w376 w377] -> w284
            tunnel: string[] [] ("array") -> [w376 w378]
            frame False {
            }
            frame True {
              n89 = Build Array (concatenate)(w378, string[] ["NO", "NO2", "NOx"] ("array")) -> (w377:string[])
            }
          }
          n90 = Delete From Array(array=w265, length=w266) -> (deleted portion=w260:string[], array with subset deleted=w264:string[])  [unwired: 1 in]
          n91 = Array Size(array=w264) -> (size(s)=w331:i32)
          n92 = property on="SO2" class="Bool (strict)"() -> ("Value"=w285:bool)  [unwired: 2 in, 2 out]
          n93 = Array Size(array=w260) -> (size(s)=w263:i32)
          n94 = Format Date/Time String(time format string (%c)="%Y%m%d %H%M", seconds (now)=w350, UTC format=FALSE) -> (date/time string=w291:string)
          n95 = for {
            N: w331 -> [_]
            tunnel: w264 -> [w717] mode=indexing
            shift-right: [w716] -> w328
            shift-left: string[] [] -> [w715]
            # "Add Parens to Units"
            n96 = Concatenate Strings(" (" ("string"), w717, ")" ("string")) -> (w714:string)
            n97 = Build Array (concatenate)(w715, w714) -> (w716:string[])
          }
          n98 = case shown="True" w285 {
            tunnel: w284 -> [w372 w374]
            tunnel: [w372 w373] -> w283
            frame False {
            }
            frame True {
              n99 = Build Array (concatenate)(w374, string[] ["SO2"] ("array")) -> (w373:string[])
            }
          }
          n100 = Array Size(array=w268) -> (size(s)=w270:i32)
          n101 = for {
            N: w263 -> [_]
            tunnel: w260 -> [w358] mode=indexing
            shift-right: [w357] -> w261
            shift-left: string[] [] -> [w356]
            # "Add Parens to Units"
            n102 = Concatenate Strings(" (" ("string"), w358, ")" ("string")) -> (w355:string)
            n103 = Build Array (concatenate)(w356, w355) -> (w357:string[])
          }
          n104 = property on="O3" class="Bool (strict)"() -> ("Value"=w282:bool)  [unwired: 2 in, 2 out]
          n105 = for {
            N: w270 -> [_]
            tunnel: w268 -> [w362] mode=indexing
            shift-right: [w361] -> w267
            shift-left: string[] [] -> [w359]
            # "Build Array of Appropriate T Units"
            n106 = case shown="10325" w362 {
              tunnel: [" (C)" " (F)" " (?)" " (K)" " (R)"] -> w360
              frame 10143 {
              }
              frame 10144 {
              }
              frame 10065, Default {
              }
              frame 10325 {
              }
              frame 10145 {
              }
            }
            n107 = Build Array (concatenate)(w359, w360) -> (w361:string[])
          }
          n108 = Path To String(path="folder path for Data (dialog if empty) 2") -> (string=w294:string)
          n109 = Concatenate Strings(w294, w295, " Gas Analyzer " ("string"), w291, ".txt" ("string")) -> (w289:string)
          "File Path for Gas Analyzer Data" <- w289
          n110 = case shown="True" w282 {
            tunnel: w283 -> [w368 w370]
            tunnel: [w368 w369] -> w278
            frame False {
            }
            frame True {
              n111 = Build Array (concatenate)(w370, string[] ["O3"] ("array")) -> (w369:string[])
            }
          }
          n112 = String To Path(string=w289) -> (path=w288:path)
          n113 = Concatenate Strings(w294, w295, w291, ".txt" ("string")) -> (w296:string)
          "File Path for PAM Data" <- w296
          n114 = Build Array (concatenate)(string[] ["", ""], w329, w328, w267, w261) -> (w324:string[])
          n115 = String To Path(string=w296) -> (path=w346:path)
          n116 = Array Size(array=w324) -> (size(s)=w325:i32)
          n117 = Build Array (concatenate)(w276, w337, w342) -> (w323:string[])
          n118 = for {
            N: w325 -> [_]
            tunnel: w324 -> [w710] mode=indexing
            tunnel: w323 -> [w711] mode=indexing
            shift-right: [w709] -> w321
            shift-left: string[] [] -> [w707]
            n119 = Concatenate Strings(w711, w710) -> (w708:string)
            n120 = Build Array (concatenate)(w707, w708) -> (w709:string[])
          }
          n121 = Build Array (concatenate)(w276, w278) -> (w277:string[])
          n122 = case shown="True" "Log PAM Data?" {
            tunnel: w321 -> [_ w730]
            tunnel: w346 -> [w727 w729]
            tunnel: [w727 w728] -> w345
            frame False {
            }
            frame True {
              w733 = TRUE  # append to file?
              # "Write Channel Names"
              # "Write Header"
              n123 = call-poly <vilib>:"Write To Spreadsheet File.vi"("delimiter (\\t)"="Delimeter", "append to file? (new file:F)"=FALSE, "2D data"="Header Information", "file path (dialog if empty)"=w729) -> ()  [unwired: 4 in, 1 out]
              n124 = local read "Delimeter"() -> (w731:string)
              n125 = call-poly <vilib>:"Write To Spreadsheet File.vi"("delimiter (\\t)"=w731, "append to file? (new file:F)"=w733, "1D data"=w730, "file path (dialog if empty)"=w729) -> ("new file path (Not A Path if cancelled)"=w728:path)  [unwired: 3 in, 1 out]
            }
          }
          n126 = case shown="True" w314 {
            tunnel: "Run Start Time" -> [_ w544]
            tunnel: w312 -> [_ w543]
            frame False {
              # "Manual"
              n127 = property on="Run In Progress?" class="Bool (strict)"("Value"=TRUE ("Run In Progress?")) -> ()  [unwired: 2 in, 2 out]
            }
            frame True {
              # "Auto"
              n128 = while {
                tunnel: w544 -> [w550]
                tunnel: w543 -> [w549]
                stop <- w548 stop-if-true
                n129 = Get Date/Time In Seconds() -> (seconds since 1Jan1904=w551:timestamp)
                n130 = Subtract(x=w551, y=w550) -> (x-y=w546:dbl)
                n131 = Greater Or Equal?(x=w551, y=w550) -> (x >= y?=w552:bool)
                n132 = Less Or Equal?(x=w546, y=w549) -> (x <= y?=w547:bool)
                n133 = And(x=w552, y=w547) -> (x .and. y?=→"Run In Progress?":bool)
                n134 = property on="Stop Button" class="Bool (strict)"() -> ("Value"=w548:bool)  [unwired: 2 in, 2 out]
              }
            }
          }
          n135 = case shown="True" "Log Thermo Data?" {
            tunnel: w288 -> [w380 w386]
            tunnel: [w380 w382] -> w279
            tunnel: w277 -> [_ w381]
            frame False {
            }
            frame True {
              # "Write Header"
              # "Write Channel Names"
              n136 = local read "Delimeter"() -> (w389:string)
              n137 = call-poly <vilib>:"Write To Spreadsheet File.vi"("delimiter (\\t)"=w389, "append to file? (new file:F)"=FALSE, "2D data"=string[][] [["Thermo Gas Analyzer Data"]], "file path (dialog if empty)"=w386) -> ("new file path (Not A Path if cancelled)"=w385:path)  [unwired: 4 in]
              n138 = local read "Delimeter"() -> (w383:string)
              n139 = call-poly <vilib>:"Write To Spreadsheet File.vi"("delimiter (\\t)"=w383, "append to file? (new file:F)"=TRUE, "1D data"=w381, "file path (dialog if empty)"=w385) -> ("new file path (Not A Path if cancelled)"=w382:path)  [unwired: 3 in, 1 out]
            }
          }
          n140 = property on="SO2 Data" class="WFChart (strict)"("History Data"=sgl[] []) -> ()  [unwired: 2 in, 2 out]
          n141 = property on="NO, NO2, NOx Data" class="WFChart (strict)"("History Data"=dbl[][] []) -> ()  [unwired: 2 in, 2 out]
          n142 = property on="O3 Data" class="WFChart (strict)"("History Data"=sgl[] []) -> ()  [unwired: 2 in, 2 out]
          n143 = Get Date/Time In Seconds() -> (seconds since 1Jan1904=w302:timestamp)
          n144 = Reciprocal(x="Frequency (Hz)") -> (1/x=w300:dbl)
          n145 = To Double Precision Float(number=w302) -> (double precision float=w299:dbl)
          n146 = property on="O3 Data" class="WFChart (strict)"("XScale.Multiplier"=w300, "XScale.Offset"=w299, "YScale.Minimum"=0.0 ("Y Scale.Range:Minimum")) -> ()  [unwired: 2 in, 2 out]
          n147 = property on="NO, NO2, NOx Data" class="WFChart (strict)"("XScale.Multiplier"=w300, "XScale.Offset"=w299, "YScale.Minimum"=0.0 ("Y Scale.Range:Minimum")) -> ()  [unwired: 2 in, 2 out]
          n148 = property on="SO2 Data" class="WFChart (strict)"("XScale.Multiplier"=w300, "XScale.Offset"=w299, "YScale.Minimum"=0.0 ("Y Scale.Range:Minimum")) -> ()  [unwired: 2 in, 2 out]
          n149 = property on="Log Thermo Data?" class="Bool (strict)"() -> ("Value"=w280:bool)  [unwired: 2 in, 2 out]
          n150 = Obtain Notifier(name (unnamed)="STOP", notification data type=FALSE, error in (no error)=errorcluster {"status"=FALSE, "code"=0, "source"=""}) -> (notifier out=w272:refnum<notifier>, error out=w271:errorcluster)  [unwired: 1 in, 1 out]
          n151 = while {
            tunnel: errorcluster {"status"=FALSE, "code"=0, "source"=""} ("Error In") -> [w400]
            tunnel: [w399] -> w281
            tunnel: "In Use? 17" -> [w396]
            tunnel: "In Use? 18" -> [w402]
            tunnel: "In Use? 17" -> [w401]
            tunnel: w300 -> [w398]
            tunnel: w280 -> [w397]
            tunnel: w279 -> [w395]
            tunnel: w272 -> [w393]
            tunnel: w271 -> [w392]
            stop <- w394 stop-if-true
            n152 = Wait on Notification(notifier=w393, timeout in ms (-1)=10, error in (no error)=w392) -> (notification=w390:bool)  [unwired: 1 in, 3 out]
            n153 = case shown="False" w390 {
              tunnel: w402 -> [w431 _]
              tunnel: w401 -> [w430 _]
              tunnel: w400 -> [w429 w541]
              tunnel: [w428 w541] -> w399
              tunnel: w398 -> [w419 _]
              tunnel: w397 -> [w417 _]
              tunnel: w396 -> [w412 _]
              tunnel: w395 -> [w405 _]
              frame False {
                n154 = case shown="True" w430 {
                  tunnel: w429 -> [w493 w503]
                  tunnel: [w493 w501] -> w424
                  tunnel: [sgl[] [] w495] -> w425
                  tunnel: w412 -> [_ w496]
                  tunnel: [sgl[] [] w494] -> w414
                  frame False {
                  }
                  frame True {
                    n155 = call "Thermo Gas Conc Read (SubVI).vi"("Error In"=w503, "Instrument"="Instrument 2") -> ("error out"=w498:errorcluster, "Data Out"=w502:T9)  [unwired: 8 in]
                    n156 = Array Size(array=w502) -> (size(s)=w499:i32)
                    n157 = property on="SO2 Data" class="WFChart (strict)"(error in=w498, "LegAutosize"=TRUE ("Legend:Autosize"), "LegNumRows"=w499) -> (error out=w497:errorcluster)  [unwired: 1 in, 1 out]
                    n158 = for {
                      N: w499 -> [_]
                      tunnel: w502 -> [w512] mode=indexing
                      shift-right: [w509] -> w501
                      shift-left: w497 -> [w508]
                      tunnel: [w507] -> w495 mode=indexing
                      i -> [w511]
                      n159 = Unbundle By Name(w512) -> ("Label"=w510:string, "Concentration"=w507:sgl)
                      n160 = property on="SO2 Data" class="WFChart (strict)"(error in=w508, "Active Plot"=w511, "Plot.Plot Name"=w510) -> (error out=w509:errorcluster)  [unwired: 1 in, 1 out]
                    }
                    n161 = case shown="True" w496 {
                      tunnel: w495 -> [_ w506]
                      tunnel: [sgl[] [] w506] -> w494
                      frame False {
                      }
                      frame True {
                      }
                    }
                  }
                }
                "SO2 Data" <- w425
                n162 = case shown="True" w431 {
                  tunnel: w429 -> [w471 w481]
                  tunnel: [w471 w475] -> w423
                  tunnel: [sgl[] [] w473] -> w413
                  tunnel: w412 -> [_ w474]
                  tunnel: [sgl[] [] w472] -> w411
                  frame False {
                  }
                  frame True {
                    n163 = call "Thermo Gas Conc Read (SubVI).vi"("Error In"=w481, "Instrument"="Instrument 3") -> ("error out"=w480:errorcluster, "Data Out"=w479:T9)  [unwired: 8 in]
                    n164 = Array Size(array=w479) -> (size(s)=w478:i32)
                    n165 = property on="O3 Data" class="WFChart (strict)"(error in=w480, "LegAutosize"=TRUE ("Legend:Autosize"), "LegNumRows"=w478) -> (error out=w476:errorcluster)  [unwired: 1 in, 1 out]
                    n166 = for {
                      N: w478 -> [_]
                      tunnel: w479 -> [w490] mode=indexing
                      tunnel: [w488] -> w473 mode=indexing
                      shift-right: [w486] -> w475
                      shift-left: w476 -> [w485]
                      i -> [w487]
                      n167 = Unbundle By Name(w490) -> ("Label"=w489:string, "Concentration"=w488:sgl)
                      n168 = property on="O3 Data" class="WFChart (strict)"(error in=w485, "Active Plot"=w487, "Plot.Plot Name"=w489) -> (error out=w486:errorcluster)  [unwired: 1 in, 1 out]
                    }
                    n169 = case shown="True" w474 {
                      tunnel: w473 -> [_ w484]
                      tunnel: [sgl[] [] w484] -> w472
                      frame False {
                      }
                      frame True {
                      }
                    }
                  }
                }
                "O3 Data" <- w413
                n170 = case shown="True" w412 {
                  tunnel: [w515 w523] -> w427
                  tunnel: w429 -> [w515 w526]
                  tunnel: [T7 [] ("Real Matrix") w517] -> w418
                  tunnel: w417 -> [_ w518]
                  tunnel: [dbl[] [] ("Real 2D Array") w516] -> w415
                  frame False {
                  }
                  frame True {
                    n171 = call "Thermo Gas Conc Read (SubVI).vi"("Error In"=w526, "Instrument"="Instrument") -> ("error out"=w520:errorcluster, "Data Out"=w525:T9)  [unwired: 8 in]
                    n172 = Array Size(array=w525) -> (size(s)=w521:i32)
                    n173 = property on="NO, NO2, NOx Data" class="WFChart (strict)"(error in=w520, "LegAutosize"=TRUE ("Legend:Autosize"), "LegNumRows"=w521) -> (error out=w519:errorcluster)  [unwired: 1 in, 1 out]
                    n174 = for {
                      N: w521 -> [_]
                      tunnel: w525 -> [w540] mode=indexing
                      shift-right: [w538] -> w517
                      shift-left: T7 [] ("Real Matrix") -> [w537]
                      shift-right: [w534] -> w523
                      shift-left: w519 -> [w533]
                      i -> [w536]
                      n175 = Unbundle By Name(w540) -> ("Label"=w535:string, "Concentration"=w539:sgl)
                      n176 = property on="NO, NO2, NOx Data" class="WFChart (strict)"(error in=w533, "Active Plot"=w536, "Plot.Plot Name"=w535) -> (error out=w534:errorcluster)  [unwired: 1 in, 1 out]
                      n177 = Build Array (concatenate)(w537, w539) -> (w538:T7)
                    }
                    n178 = case shown="True" w518 {
                      tunnel: w517 -> [_ w532]
                      tunnel: [dbl[] [] ("Real 2D Array") w529] -> w516
                      frame False {
                      }
                      frame True {
                        n179 = call-poly <vilib>:"Matrix To Array.vi"("Real Matrix"=w532) -> ("Real 2D Array"=w531:dbl[][])
                        n180 = Index Array(array=w531, index (row)=0 ("disabled index (col)")) -> (element=w529:dbl[])  [unwired: 1 in]
                      }
                    }
                  }
                }
                "NO, NO2, NOx Data" <- w418
                n181 = Multiply(x=w419, y=1000.0) -> (x*y=w420:dbl)
                n182 = Wait Until Next ms Multiple(millisecond multiple=w420) -> ()  [unwired: 1 out]
                n183 = case shown="Error" w427 {
                  selector: w427 -> [w463 w468]
                  tunnel: [w463 w467] -> w426
                  frame No Error {
                  }
                  frame Error {
                    w464 = T8 0 items=["no dialog", "OK message", "continue or stop message", "OK message + warnings", "continue/stop + warnings"] ("type of dialog (OK msg:1)")
                    n184 = call <vilib>:"General Error Handler.vi"("[error code] (0)"=5011, "[error source] (\" \")"="NOx Charting" ("[error source] (\" \")"), "type of dialog (OK msg:1)"=w464, "error in (no error)"=w468) -> ("error out"=w467:errorcluster)  [unwired: 7 in, 4 out]
                  }
                }
                n185 = case shown="Error" w424 {
                  selector: w424 -> [w457 w462]
                  tunnel: [w457 w461] -> w416
                  frame No Error {
                  }
                  frame Error {
                    w458 = T8 0 items=["no dialog", "OK message", "continue or stop message", "OK message + warnings", "continue/stop + warnings"] ("type of dialog (OK msg:1)")
                    n186 = call <vilib>:"General Error Handler.vi"("[error code] (0)"=5011, "[error source] (\" \")"="SO2 Charting" ("[error source] (\" \")"), "type of dialog (OK msg:1)"=w458, "error in (no error)"=w462) -> ("error out"=w461:errorcluster)  [unwired: 7 in, 4 out]
                  }
                }
                n187 = case shown="Error" w423 {
                  selector: w423 -> [w451 w456]
                  tunnel: [w451 w455] -> w422
                  frame No Error {
                  }
                  frame Error {
                    w452 = T8 0 items=["no dialog", "OK message", "continue or stop message", "OK message + warnings", "continue/stop + warnings"] ("type of dialog (OK msg:1)")
                    n188 = call <vilib>:"General Error Handler.vi"("[error code] (0)"=5011, "[error source] (\" \")"="O3 Charting" ("[error source] (\" \")"), "type of dialog (OK msg:1)"=w452, "error in (no error)"=w456) -> ("error out"=w455:errorcluster)  [unwired: 7 in, 4 out]
                  }
                }
                n189 = Build Array (concatenate)(w415, w414, w411) -> (w410:dbl[])
                n190 = Merge Errors(w426, w416, w422) -> (w428:errorcluster)
                n191 = Get Date/Time In Seconds() -> (seconds since 1Jan1904=w408:timestamp)
                n192 = property on="Log Thermo Data?" class="Bool (strict)"() -> ("Value"=w406:bool)  [unwired: 2 in, 2 out]
                n193 = Format Date/Time String(seconds (now)=w408, UTC format=FALSE ("to UTC (F)")) -> (date/time string=w404:string)  [unwired: 1 in]
                n194 = Format Date/Time String(seconds (now)=w408, UTC format=TRUE ("to UTC (F)")) -> (date/time string=w403:string)  [unwired: 1 in]
                n195 = case shown="True" w406 {
                  tunnel: w410 -> [_ w441]
                  tunnel: w405 -> [w432 w436]
                  tunnel: w404 -> [_ w435]
                  tunnel: w403 -> [_ w434]
                  tunnel: [w432 w433] -> _
                  frame False {
                  }
                  frame True {
                    n196 = Array Size(array=w441) -> (size(s)=w442:i32)
                    n197 = for {
                      N: w442 -> [_]
                      shift-right: [w449] -> w440
                      shift-left: string[] [] -> [w447]
                      tunnel: w441 -> [w444] mode=indexing
                      i -> [w450]
                      n198 = Format Value(string ("")="", format string="%.3f", value (0)=w444) -> (output string=w448:string)
                      n199 = Insert Into Array(array=w447, index=w450, new element=w448) -> (w449:string[])
                    }
                    n200 = local read "Delimeter"() -> (w437:string)
                    n201 = Build Array (concatenate)(w435, w434, w440) -> (w439:string[])
                    n202 = call-poly <vilib>:"Write To Spreadsheet File.vi"("delimiter (\\t)"=w437, "append to file? (new file:F)"=TRUE, "1D data"=w439, "file path (dialog if empty)"=w436) -> ("new file path (Not A Path if cancelled)"=w433:path)  [unwired: 3 in, 1 out]
                  }
                }
              }
              frame True {
                # "This case will execute if there is an error in the notifier, otherwise it should never be seen!"
              }
            }
            n203 = Or(x=w399, y=w390) -> (x .or. y?=w394:bool)
          }
          n204 = while {
            tunnel: w341 -> [w793]
            tunnel: w340 -> [w794]
            tunnel: [w822] -> w336
            tunnel: w343 -> [w781]
            tunnel: w344 -> [w819]
            tunnel: [w737] -> w318
            tunnel: w338 -> [w796]
            tunnel: w339 -> [w797]
            tunnel: "Run Start Time" -> [w812]
            tunnel: w345 -> [w809]
            tunnel: w335 -> [w770]
            tunnel: w334 -> [w777]
            shift-right: [w745] -> _
            shift-left: _ -> [w749]
            shift-right: [w742] -> _
            shift-left: 0.0 -> [w746]
            tunnel: w272 -> [w739]
            tunnel: w271 -> [w738]
            stop <- w736 stop-if-true
            # "Filter Advantech TC Data"
            # "Sets the Data Logging Frequency"
            # "Add in case structure here to shut everything off if LED goes off"
            # "RHT T Probes\nRHT RH Probes\nMFC Probes\nNI TC Probes\nPressure Trans."
            # "NI AI"
            # "Advantech"
            n205 = Get Date/Time In Seconds() -> (seconds since 1Jan1904=w811:timestamp)
            n206 = Subtract(x=w811, y=w812) -> (x-y=w764:dbl)
            n207 = Greater Or Equal?(x=w811, y=w812) -> (x >= y?=w767:bool)
            n208 = call-poly <vilib>:"DAQmx Read.vi"("task/channels in"=w794, "error in"=w793) -> ("task out"=w822:refnum<k21>, "data"=w743:waveform(dbl)[], "error out"=w802:errorcluster)  [unwired: 11 in]
            n209 = Divide(x=w764, y=60.0) -> (x/y=→"Elapsed Time (min)":dbl)
            n210 = call "DAQNavi Assistant"("error in(no error)"=w802) -> ("error out"=w737:errorcluster, "data out(DDT)"=w741:dynamicdata)  [unwired: 17 in]
            n211 = call "Convert from Dynamic Data4"("Dynamic Data Type"=w741) -> ("Array"=w744:dbl[])  [unwired: 3 in]
            n212 = call "Convert from Dynamic Data5"("Dynamic Data Type"=w749) -> ("Array"=w748:dbl[])  [unwired: 3 in]
            n213 = Array Size(array=w744) -> (size(s)=w755:i32)
            n214 = call "Convert from Dynamic Data6"("Dynamic Data Type"=w741) -> ()  [unwired: 3 in, 1 out]
            n215 = Initialize Array(1.15 ("element"), w755) -> (w762:dbl[])
            n216 = Initialize Array(0.85 ("element"), w755) -> (w761:dbl[])
            n217 = Multiply(x=w762, y=w748) -> (x*y=w753:dbl[])
            n218 = Multiply(x=w761, y=w748) -> (x*y=w752:dbl[])
            n219 = Greater?(x=w744, y=w753) -> (0:w760:bool[])
            n220 = Less?(x=w744, y=w752) -> (x < y?=w747:bool[])
            n221 = Or(x=w760, y=w747) -> (x .or. y?=w751:bool[])
            n222 = Boolean To (0,1)(Boolean=w751) -> (0, 1=w750:i16[])
            n223 = Add Array Elements(numeric array=w750) -> (sum=w759:i16)
            n224 = Greater?(x=w759, y=i16 0) -> (0:w754:bool)
            n225 = case shown="True" w754 {
              tunnel: w741 -> [w828 _]
              tunnel: [w828 w831] -> w745
              tunnel: w749 -> [_ w831]
              tunnel: [w827 w830] -> w742
              tunnel: w746 -> [w827 w829]
              frame False {
              }
              frame True {
                n226 = Increment(x=w829) -> (x+1=w830:dbl)
              }
            }
            "Bad Advantech Data Points" <- w742
            n227 = Split 1D Array(array=w743, index=w797) -> (first subarray=w815:waveform(dbl)[], second subarray=w824:waveform(dbl)[])
            n228 = Array Size(array=w777) -> (size(s)=w774:i32)
            n229 = Split 1D Array(array=w824, index=w796) -> (first subarray=w814:waveform(dbl)[], second subarray=w823:waveform(dbl)[])
            "Relative Humidity Data" <- w814
            n230 = Split 1D Array(array=w823, index=w819) -> (first subarray=w813:waveform(dbl)[], second subarray=w780:waveform(dbl)[])
            n231 = Split 1D Array(array=w780, index=w781) -> (first subarray=w779:waveform(dbl)[], second subarray=w778:waveform(dbl)[])
            n232 = for {
              N: w774 -> [_]
              tunnel: w778 -> [w841] mode=indexing
              tunnel: w777 -> [w844] mode=indexing
              shift-right: [w835] -> w772
              shift-left: waveform(dbl)[] [] -> [w834]
              # "First, exponentiate and solve in terms of Torr by P[torr] = exp((Volts-6)/0.4343)"
              n233 = Unbundle By Name(w844) -> ("Label"=w832:string, "Units Num"=w843:i32)
              n234 = To Unsigned Word Integer(number=w843) -> (unsigned 16bit integer=w842:u16)
              n235 = Subtract(x=w841, y=6.0) -> (x-y=w839:waveform(dbl))
              n236 = Divide(x=w839, y=0.4343) -> (x/y=w837:waveform(dbl))
              n237 = Exponential(1:w837) -> (0:w836:waveform(dbl))
              n238 = case shown="0, Default" w842 {
                tunnel: w832 -> [_ _ _ _]
                tunnel: w836 -> [w845 w848 w851 w854]
                tunnel: [w845 w847 w850 w853] -> w833
                frame 0, Default {
                  # "Torr"
                }
                frame 1 {
                  # "Psia"
                  n239 = Multiply(x=w848, y=0.0193396) -> (x*y=w847:waveform(dbl))
                }
                frame 2 {
                  # "Bar"
                  n240 = Multiply(x=w851, y=0.001333) -> (x*y=w850:waveform(dbl))
                }
                frame 3 {
                  # "kPa"
                  n241 = Multiply(x=w854, y=0.1333) -> (x*y=w853:waveform(dbl))
                }
              }
              n242 = Build Array (concatenate)(w834, w833) -> (w835:waveform(dbl)[])
            }
            n243 = call "Convert from Dynamic Data3"("Dynamic Data Type"=w745) -> ("Array"=w799:dbl[])  [unwired: 3 in]
            n244 = Merge Signals(w745, w815, w779) -> (w803:dynamicdata)
            "Temperature Data" <- w803
            n245 = call "Convert from Dynamic Data"("Dynamic Data Type"=w803) -> ("Array"=→"TC Values Readings":dbl[])  [unwired: 3 in]
            n246 = Array Size(array=w743) -> (size(s)=w771:i32)
            n247 = Subtract(x=w771, y=w770) -> (x-y=w768:i32)
            n248 = Replace Array Subset(array=w743, new element=w772, index=w768) -> (w769:waveform(dbl)[])
            n249 = Index Array(array=w772, index=0) -> (element=w773:waveform(dbl))
            "Pressure Transducer" <- w773
            n250 = Build Array (concatenate)(w799, w769) -> (w798:dbl[])
            n251 = Merge Signals(w814, w813, w773) -> (w820:dynamicdata)
            n252 = Split Signals(w813) -> (→"N2 Reading (LPM)":dynamicdata, →"O2 Reading (LPM)":dynamicdata, →"NOx Reading (LPM) 3":dynamicdata, →"VOC Reading (LPM)":dynamicdata)  [unwired: 4 in]
            n253 = call "Convert from Dynamic Data2"("Dynamic Data Type"=w820) -> ("Array"=→"RH Values":dbl[])  [unwired: 3 in]
            n254 = Array Size(array=w798) -> (size(s)=w801:i32)
            n255 = for {
              N: w801 -> [_]
              shift-right: [w861] -> w792
              shift-left: string[] [] -> [w859]
              tunnel: w798 -> [w855] mode=indexing
              i -> [w862]
              n256 = To Double Precision Float(number=w855) -> (double precision float=w858:dbl)
              n257 = Format Value(string ("")="", format string="%.3f", value (0)=w858) -> (output string=w860:string)
              n258 = Insert Into Array(array=w859, index=w862, new element=w860) -> (w861:string[])
            }
            n259 = local read "Log PAM Data?"() -> (w791:bool)
            n260 = call "Elapsed Time"("Time Target (s)"="Data Logging Interval (s)", "Reset"=FALSE, "Auto Reset"=TRUE, "Set Start Time (s)"=0.0) -> ("Time has Elapsed"=w790:bool)  [unwired: 8 in, 7 out]
            n261 = Get Date/Time In Seconds() -> (seconds since 1Jan1904=w807:timestamp)
            n262 = Divide(x=1.0, y="Sampling Frequency (Hz)") -> (x/y=w784:dbl)
            n263 = Multiply(x=1000.0, y=w784) -> (x*y=w782:dbl)
            n264 = And(x=w790, y=w791) -> (x .and. y?=w788:bool)
            n265 = Format Date/Time String(seconds (now)=w807, UTC format=FALSE ("to UTC (F)")) -> (date/time string=w804:string)  [unwired: 1 in]
            n266 = Format Date/Time String(seconds (now)=w807, UTC format=TRUE ("to UTC (F)")) -> (date/time string=w805:string)  [unwired: 1 in]
            n267 = Wait Until Next ms Multiple(millisecond multiple=w782) -> ()  [unwired: 1 out]
            n268 = case shown="True" w788 {
              tunnel: w809 -> [w863 w871]
              tunnel: [w863 w870] -> _
              tunnel: w805 -> [_ w866]
              tunnel: w804 -> [_ w865]
              tunnel: w792 -> [_ w864]
              frame False {
              }
              frame True {
                n269 = Build Array (concatenate)(w865, w866, w864) -> (w867:string[])
                n270 = local read "Delimeter"() -> (w869:string)
                n271 = call-poly <vilib>:"Write To Spreadsheet File.vi"("delimiter (\\t)"=w869, "append to file? (new file:F)"=TRUE, "1D data"=w867, "file path (dialog if empty)"=w871) -> ("new file path (Not A Path if cancelled)"=w870:path)  [unwired: 3 in, 1 out]
              }
            }
            n272 = Or(x=w737, y="Stop Button") -> (x .or. y?=w736:bool)
            n273 = Send Notification(notification=w736, notifier=w739, error in (no error)=w738) -> ()  [unwired: 2 out]
            n274 = Not(x=w736) -> (.not. x?=w810:bool)
            n275 = And(x=w767, y=w810) -> ()  [unwired: 1 out]
          }
          n276 = while {
            tunnel: w320 -> [w569]
            tunnel: "Run Start Time" -> [w562]
            tunnel: [w567] -> w319
            tunnel: [w556] -> w316
            tunnel: w314 -> [w564]
            tunnel: w315 -> [w565]
            tunnel: w272 -> [w560]
            tunnel: w271 -> [w559]
            tunnel: [w558] -> _
            tunnel: [w557] -> _
            stop <- w555 stop-if-true
            n277 = Get Date/Time In Seconds() -> (seconds since 1Jan1904=w563:timestamp)
            n278 = Greater Or Equal?(x=w563, y=w562) -> (x >= y?=w561:bool)
            n279 = Wait on Notification(notifier=w560, timeout in ms (-1)=200, error in (no error)=w559) -> (notifier out=w558:refnum<notifier>, notification=w554:bool, error out=w557:errorcluster)  [unwired: 1 in, 1 out]
            n280 = Not(x=w564) -> (.not. x?=→"Manual":bool)
            n281 = case shown="False" w564 {
              tunnel: w569 -> [w576 w597]
              tunnel: [w578 w596] -> w567
              tunnel: [w572 w595] -> w556
              tunnel: errorcluster {"status"=FALSE, "code"=0, "source"=""} ("error in") -> [w577 w581]
              tunnel: w561 -> [_ w580]
              tunnel: w565 -> [_ w582]
              tunnel: w554 -> [_ w579]
              frame False {
                # "FALSE: Manual mode is selected\nThe user can alter the flows throughout a run by using the scales on the front diagram"
                n282 = Build Array("N2 Control (LPM)", "O2 Control (LPM)", "NOx Control (LPM)", "VOC Control (LPM)") -> (w575:dbl[])
                n283 = call-poly <vilib>:"DAQmx Write.vi"("task/channels in"=w576, "data"=w575, "error in"=w577) -> ("task out"=w578:refnum<k21>, "error out"=w572:errorcluster)  [unwired: 10 in, 1 out]
              }
              frame True {
                # "TRUE: AUTO Mode is selected. Sequence files must be in place"
                n284 = Array Size(array=w582) -> (size(s)=w594:i32)
                n285 = for {
                  N: w594 -> [_]
                  tunnel: w582 -> [w616] mode=indexing
                  shift-right: [w614] -> _
                  shift-left: string[] [] -> [w613]
                  shift-right: [w611] -> w587
                  shift-left: dbl[] [] -> [w610]
                  shift-right: [w608] -> w586
                  shift-left: dbl[] [] -> [w607]
                  shift-right: [w605] -> w585
                  shift-left: dbl[] [] -> [w604]
                  shift-right: [w602] -> w584
                  shift-left: dbl[] [] -> [w601]
                  shift-right: [w599] -> w583
                  shift-left: dbl[] [] -> [w598]
                  n286 = Unbundle By Name(w616) -> ("Label"=w615:string, "Time"=w612:dbl, "SP N2"=w609:dbl, "SP O2"=w606:dbl, "SP NOx"=w603:dbl, "SP VOC"=w600:dbl)
                  n287 = Build Array (concatenate)(w613, w615) -> (w614:string[])
                  n288 = Build Array (concatenate)(w610, w612) -> (w611:dbl[])
                  n289 = Build Array (concatenate)(w607, w609) -> (w608:dbl[])
                  n290 = Build Array (concatenate)(w604, w606) -> (w605:dbl[])
                  n291 = Build Array (concatenate)(w601, w603) -> (w602:dbl[])
                  n292 = Build Array (concatenate)(w598, w600) -> (w599:dbl[])
                }
                n293 = case shown="True" w580 {
                  tunnel: w597 -> [w620 w635]
                  tunnel: [w619 w630] -> w596
                  tunnel: [w618 w629] -> w595
                  tunnel: w581 -> [w617 w637]
                  tunnel: w582 -> [_ w638]
                  tunnel: w587 -> [_ w636]
                  tunnel: w586 -> [_ w634]
                  tunnel: w585 -> [_ w633]
                  tunnel: w584 -> [_ w632]
                  tunnel: w583 -> [_ w631]
                  tunnel: w579 -> [_ w626]
                  frame False {
                    # "FALSE: Auto mode is in place, but the start time has not been reached"
                    n294 = Build Array(0.0 ("element"), 0.0 ("element"), 0.0 ("element"), 0.0 ("element")) -> (w621:dbl[])
                    n295 = call-poly <vilib>:"DAQmx Write.vi"("task/channels in"=w620, "data"=w621, "error in"=w617) -> ("task out"=w619:refnum<k21>, "error out"=w618:errorcluster)  [unwired: 10 in, 1 out]
                  }
                  frame True {
                    # "TRUE: Start time has been reached. Auto mode is in place. The experiment runs per Sequence file"
                    n296 = Array Size(array=w638) -> (size(s)=w627:i32)
                    n297 = for {
                      N: w627 -> [_]
                      tunnel: 0.0 ("Set Start Time (s)") -> [w655]
                      shift-right: [w646] -> w629
                      shift-left: w637 -> [w654]
                      tunnel: w636 -> [w653] mode=indexing
                      tunnel: w631 -> [w649] mode=indexing
                      tunnel: w632 -> [w650] mode=indexing
                      tunnel: w633 -> [w651] mode=indexing
                      tunnel: w634 -> [w652] mode=indexing
                      tunnel: w635 -> [w648]
                      tunnel: [w647] -> w630
                      tunnel: w634 -> [w645]
                      tunnel: w633 -> [w644]
                      tunnel: w632 -> [w643]
                      tunnel: w631 -> [w642]
                      tunnel: w627 -> [_]
                      tunnel: w626 -> [w640]
                      tunnel: w626 -> [w639]
                      i -> [w641]
                      stop <- w640 stop-if-true
                      n298 = while {
                        tunnel: w655 -> [w675]
                        tunnel: w654 -> [w674]
                        tunnel: w653 -> [w673]
                        tunnel: w652 -> [w672]
                        tunnel: w651 -> [w671]
                        tunnel: w650 -> [w670]
                        tunnel: w649 -> [w669]
                        tunnel: w648 -> [w668]
                        tunnel: [w667] -> w647
                        tunnel: [w666] -> w646
                        tunnel: w641 -> [w663]
                        tunnel: w645 -> [w662]
                        tunnel: w644 -> [w661]
                        tunnel: w643 -> [w660]
                        tunnel: w642 -> [w659]
                        tunnel: [w658] -> _
                        tunnel: w639 -> [w656]
                        stop <- w657 stop-if-true
                        n299 = call "Elapsed Time3"("Time Target (s)"=w673, "Reset"=FALSE, "Auto Reset"=FALSE, "error in (no error)"=w674, "Set Start Time (s)"=w675) -> ("Time has Elapsed"=w658:bool, "error out"=w665:errorcluster)  [unwired: 7 in, 6 out]
                        n300 = Or(x=w656, y=w658) -> (x .or. y?=w657:bool)
                        n301 = case shown="False" w658 {
                          tunnel: w672 -> [_ w706]
                          tunnel: w671 -> [_ w705]
                          tunnel: w670 -> [_ w704]
                          tunnel: w669 -> [_ w703]
                          tunnel: [w684 w702] -> w664
                          tunnel: w663 -> [w679 _]
                          tunnel: w662 -> [w683 _]
                          tunnel: w661 -> [w682 _]
                          tunnel: w660 -> [w681 _]
                          tunnel: w659 -> [w680 _]
                          frame False {
                            n302 = Equal To 0?(x=w679) -> (x = 0?=w685:bool)
                            n303 = case shown="False" w685 {
                              tunnel: [w691 w699] -> w684
                              tunnel: w683 -> [w696 _]
                              tunnel: w682 -> [w690 _]
                              tunnel: w681 -> [w689 _]
                              tunnel: w680 -> [w688 _]
                              tunnel: w679 -> [w687 _]
                              frame False {
                                n304 = Decrement(x=w687) -> (x-1=w686:i32)
                                n305 = Index Array(array=w696, index=w686) -> (element=w695:dbl)
                                n306 = Index Array(array=w690, index=w686) -> (element=w694:dbl)
                                n307 = Index Array(array=w689, index=w686) -> (element=w693:dbl)
                                n308 = Index Array(array=w688, index=w686) -> (element=w692:dbl)
                                n309 = Build Array(w695, w694, w693, w692) -> (w691:dbl[])
                              }
                              frame True {
                                n310 = Build Array(0, 0, 0 ("element"), 0 ("element")) -> (w699:i32[])
                              }
                            }
                            n311 = Wait (ms)(milliseconds to wait=u32 5) -> ()  [unwired: 1 out]
                          }
                          frame True {
                            n312 = Build Array(w706, w705, w704, w703) -> (w702:dbl[])
                          }
                        }
                        n313 = call-poly <vilib>:"DAQmx Write.vi"("task/channels in"=w668, "data"=w664, "error in"=w665) -> ("task out"=w667:refnum<k21>, "error out"=w666:errorcluster)  [unwired: 10 in, 1 out]
                      }
                    }
                  }
                }
              }
            }
            n314 = Or(x=w556, y=w554) -> (x .or. y?=w555:bool)
            "Auto" <- w564
          }
          n315 = Merge Errors(w318, w316, w281) -> (w317:errorcluster)
        }
        frame Error {
        }
      }
      n316 = call <vilib>:"DAQmx Clear Task.vi"("task in"=w126, "error in"=w127) -> ("error out"=w148:errorcluster)  [unwired: 13 in]
      n317 = call <vilib>:"DAQmx Clear Task.vi"("task in"=w174, "error in"=w148) -> ("error out"=w203:errorcluster)  [unwired: 13 in]
    }
    frame Error {
    }
  }
  n318 = call <vilib>:"General Error Handler.vi"("[user-defined codes]"=i32[] [5003, 5004, 5005, 5006, 5007, 5008, 5009, 5010, 5011], "[user-defined descriptions]"=string[] ["There is an error with the DAQ configuration. Check to make sure there are an equal number of Labels, Channels, and Boolean ON/OFF switches set.", "There is an error with the labels for either a MFC, RHT Probe, or TC. One or more of the instruments does not have an appropriate label. Please check them and try again.", "There is an error with one of the setup SubVI's. Please check to make sure everything is okidokie.", "There is an error with the Display Values SubVI. You may as well give up, because this thing is ugly. It's probably going to take three days to fix...", "There is an error with the MFC Sequence file. It is most likely an invalid Flow rate. The most likely error is either a flow rate out of range or a poorly chosen scale.", "There is an error with the PID Program. Check to make sure everything is set up correctly in the Sub VI.", "", "There is an error in the Thermo Gas Conc Read (SubVI).vi. Please check to make sure everything is configured correctly.", "There is an error with the charting of the Thermoscientific gas analyzers. Please check to make sure everything is configured correctly."], "error in (no error)"=w89) -> ("error out"=→"Error Out":errorcluster)  [unwired: 8 in, 4 out]
  "Scale for N2 MFC 2" <- "Scale for N2 MFC"
  "N2 MFC 2" <- "N2 MFC"
  "Scale for O2 MFC 2" <- "Scale for O2 MFC"
  "O2 MFC 2" <- "O2 MFC"
  "Scale for NOx MFC 2" <- "Scale for NOx MFC"
  "NOx MFC 2" <- "NOx MFC"
  "Scale for VOC MFC 2" <- "Scale for VOC MFC"
  "VOC MFC 2" <- "VOC MFC"
